vi "Write Sim. Command .vi"(8 "error in (no error)":errorcluster, 10 "Sim. Command":variant, 11 "Simulated uC in":refnum<class "Simulated uC.lvclass">) -> (0 "error out":errorcluster, 3 "Simulated uC out":refnum<class "Simulated uC.lvclass">)   [LabVIEW 2019, in "Simulated uC.lvclass"]
uses:
  Simulated uC.lvclass
  Simulated uC.lvclass/Simulated uC.ctl
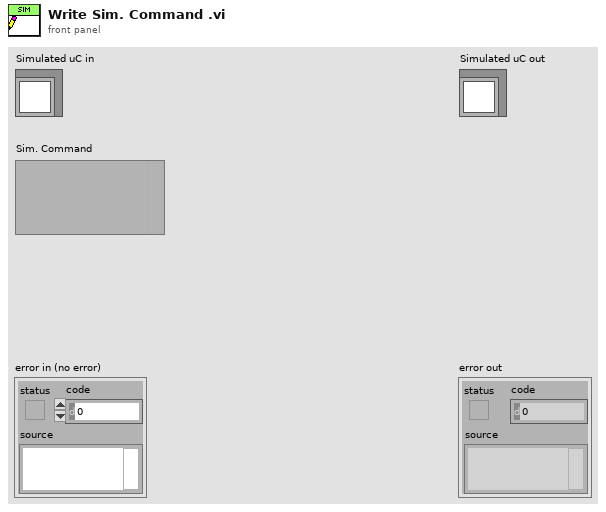
[diagram p1: front panel]
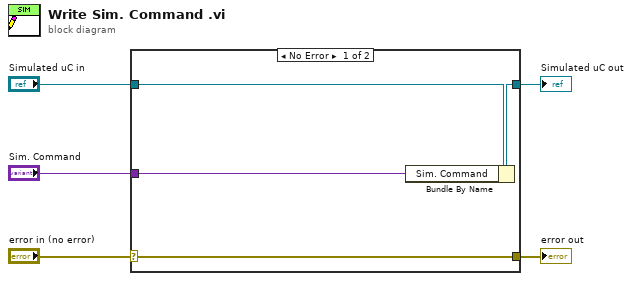
[diagram p0: block diagram]
diagram:
  n1 = case shown="No Error" "error in (no error)" {
    selector: "error in (no error)" -> [w9 w10]
    tunnel: [w9 w10] -> w4
    tunnel: [w7 w11] -> w2
    tunnel: "Simulated uC in" -> [w8 w11]
    tunnel: "Sim. Command" -> [w6 _]
    frame No Error {
      n2 = Bundle By Name(cluster=w8, "Sim. Command"=w6) -> (w7:refnum<class "Simulated uC.lvclass">)
    }
    frame Error {
    }
  }
  "error out" <- w4
  "Simulated uC out" <- w2
